vi "microFPGA_laser_mode_addr_0_ctrl.vi"(0 "VISA resource name":refnum<visa-resource-name>, 1 "laser channel":u16(ring)=3 items=["channel No 0", "channel No 1", "channel No 2", "channel No 3", "channel No 4", "channel No 5", "channel No 6", "channel No 7"], 2 "write or read":u16(ring) items=["read", "write"], 5 "Laser_mode_WRITE":u16(ring) items=["OFF", "ON", "RISING", "FALLING", "FOLLOW"], 11 "error in (no error)":errorcluster) -> (4 "VISA resource name 2":refnum<visa-resource-name>, 6 "Laser_mode_READ":u16(ring) items=["OFF", "ON", "RISING", "FALLING", "FOLLOW"], 8 "value write confirm":bool, 10 "abort_wrong_input":bool, 15 "error out":errorcluster)   [LabVIEW 2018]
panel:
  out "mode read string answer":string
  out "mode read string":string
  out "mode write string":string
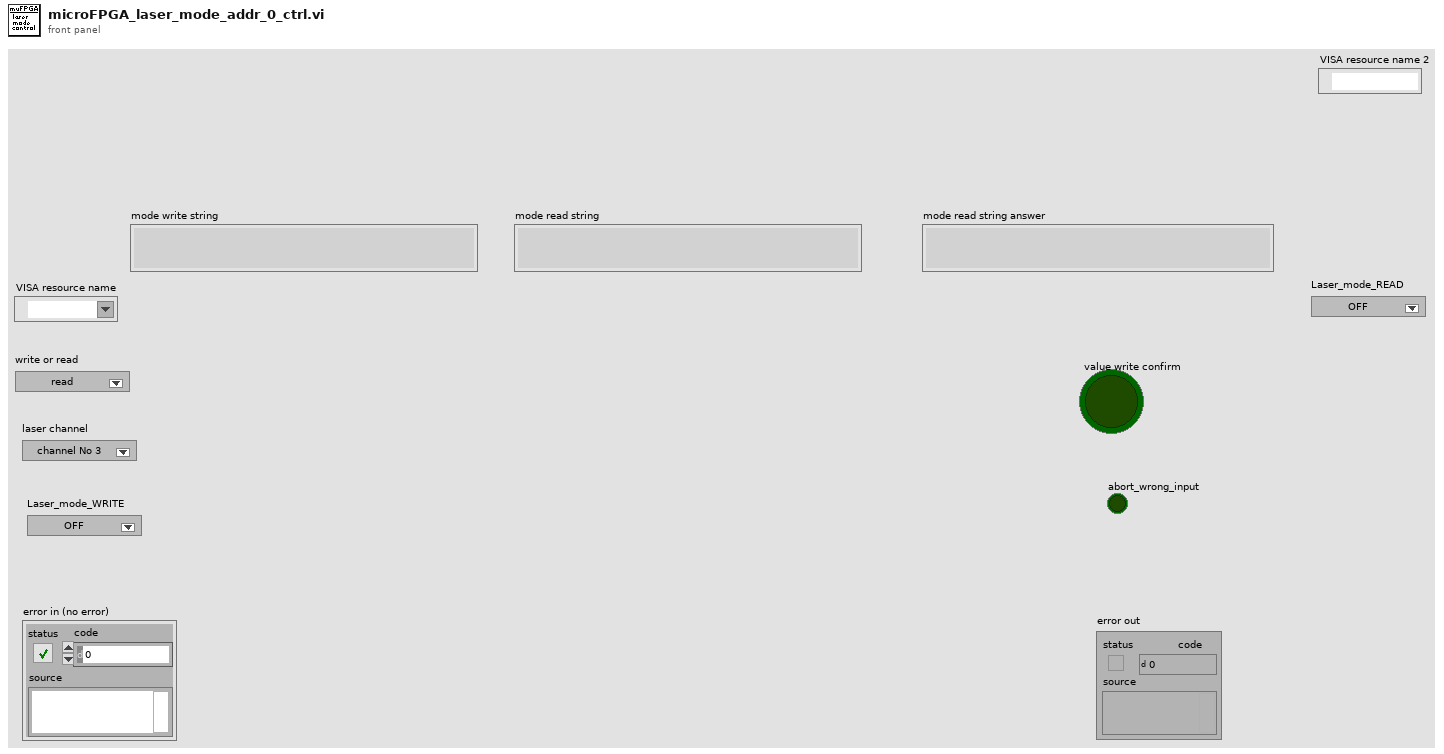
[diagram p1: front panel]
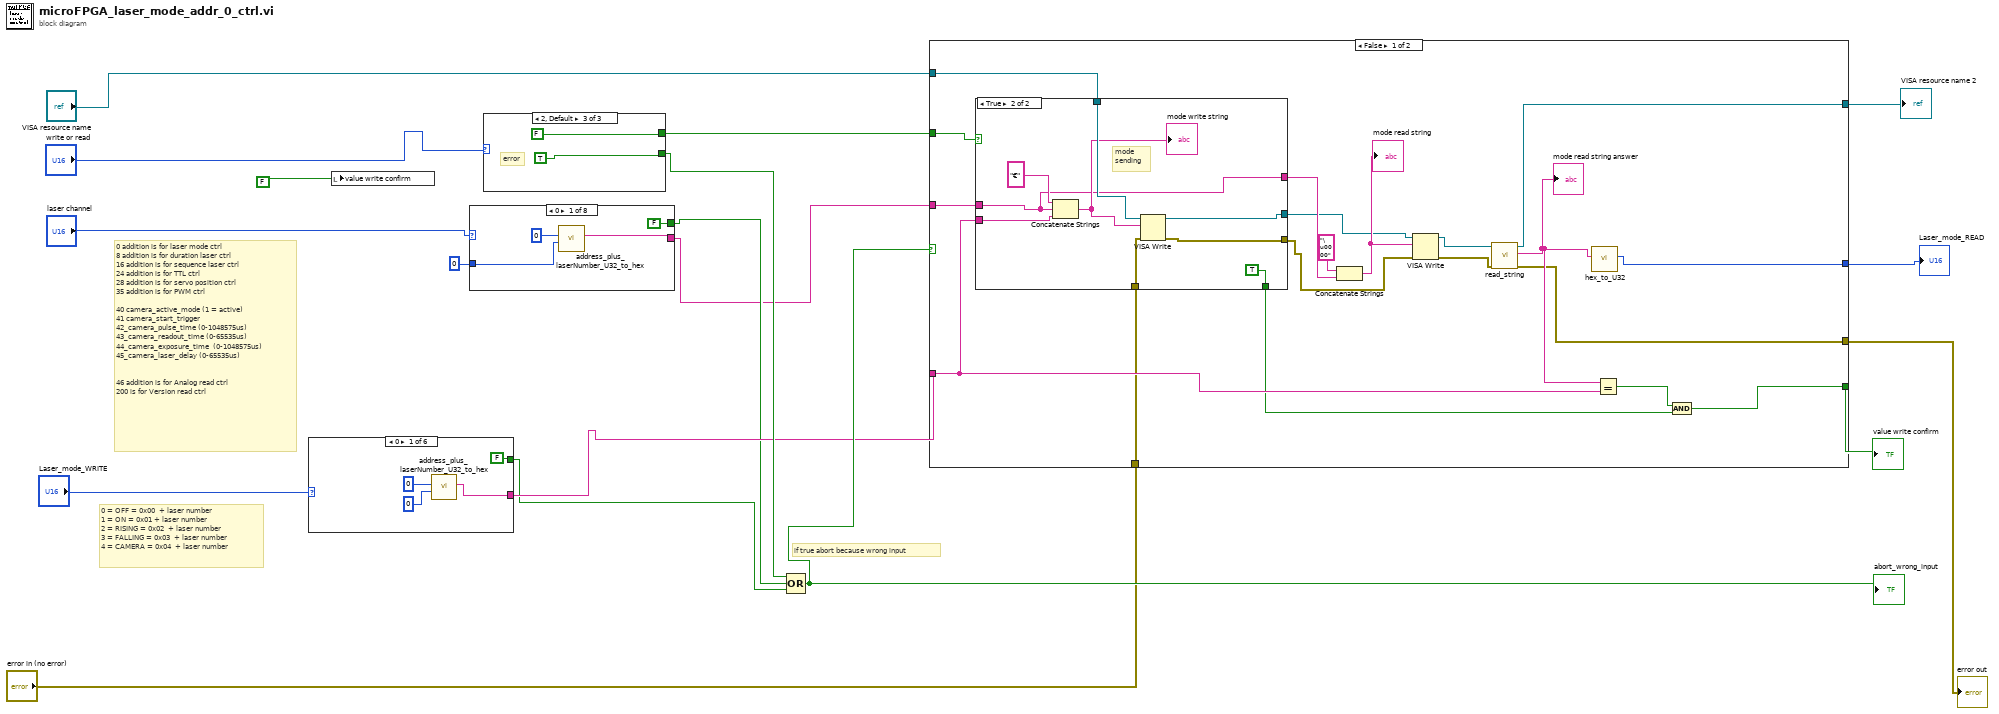
[diagram p0: block diagram]
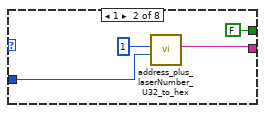
[diagram p2: hidden frame]
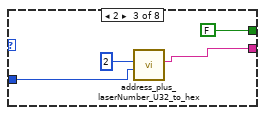
[diagram p3: hidden frame]
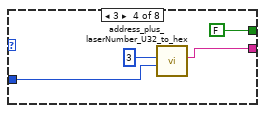
[diagram p4: hidden frame]
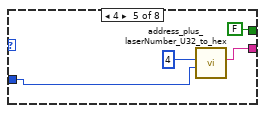
[diagram p5: hidden frame]
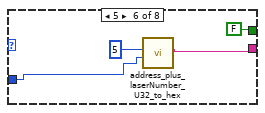
[diagram p6: hidden frame]
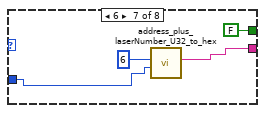
[diagram p7: hidden frame]
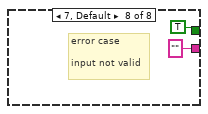
[diagram p8: hidden frame]
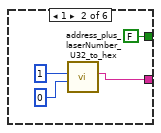
[diagram p9: hidden frame]
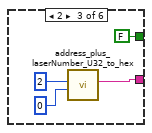
[diagram p10: hidden frame]
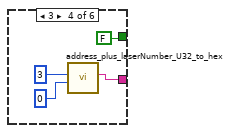
[diagram p11: hidden frame]
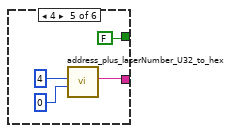
[diagram p12: hidden frame]
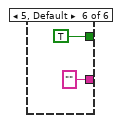
[diagram p13: hidden frame]
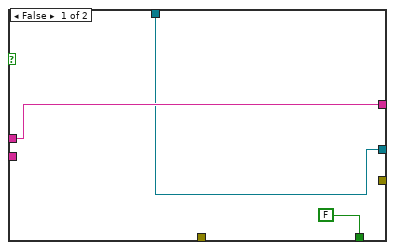
[diagram p14: hidden frame]
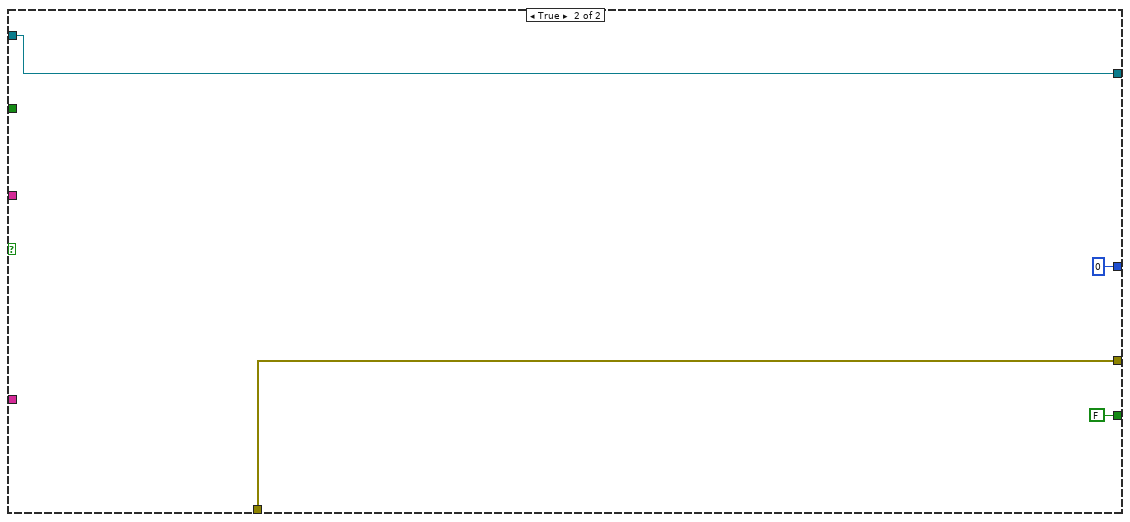
[diagram p15: hidden frame]
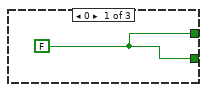
[diagram p16: hidden frame]
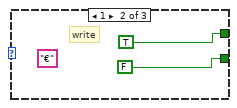
[diagram p17: hidden frame]
diagram:
  # "0 addition is for laser mode ctrl\n8 addition is for duration laser ctrl\n16 addition is for sequence laser ctrl\n24 addition is for TTL ctrl\n28 addition is for servo position ctrl\n35 addition is for PWM ctrl\n\n40 camera_active_mode (1 = active) \n41 camera_start_trigger\n42_camera_pulse_time (0-1048575us)\n43_camera_readout_time (0-65535us)\n44_camera_exposure_time  (0-1048575us)\n45_camera_laser_delay (0-65535us)\n\n\n46 addition is for Analog read ctrl\n200 is for Version read ctrl"
  # "0 = OFF = 0x00  + laser number\n1 = ON = 0x01 + laser number\n2 = RISING = 0x02  + laser number\n3 = FALLING = 0x03  + laser number\n4 = CAMERA = 0x04  + laser number"
  # "if true abort because wrong input"
  n1 = case shown="0" "Laser_mode_WRITE" {
    tunnel: [w19 w24 w28 w32 w36 "" ("string 5")] -> w7
    tunnel: [FALSE FALSE FALSE FALSE FALSE TRUE] -> w6
    frame 0 {
      n2 = call "address_plus_laserNumber_U32_to_hex.vi"("adress offset"=u32 0, "y 3"=u32 0) -> ("string 5"=w19:string)  [unwired: 8 in]
    }
    frame 1 {
      n3 = call "address_plus_laserNumber_U32_to_hex.vi"("adress offset"=u32 0, "y 3"=u32 1) -> ("string 5"=w24:string)  [unwired: 8 in]
    }
    frame 2 {
      n4 = call "address_plus_laserNumber_U32_to_hex.vi"("adress offset"=u32 0, "y 3"=u32 2) -> ("string 5"=w28:string)  [unwired: 8 in]
    }
    frame 3 {
      n5 = call "address_plus_laserNumber_U32_to_hex.vi"("adress offset"=u32 0, "y 3"=u32 3) -> ("string 5"=w32:string)  [unwired: 8 in]
    }
    frame 4 {
      n6 = call "address_plus_laserNumber_U32_to_hex.vi"("adress offset"=u32 0, "y 3"=u32 4) -> ("string 5"=w36:string)  [unwired: 8 in]
    }
    frame 5, Default {
    }
  }
  n7 = local write "value write confirm"(FALSE ("value confirm")) -> ()
  n8 = case shown="0" "laser channel" {
    tunnel: [w42 w46 w50 w54 w58 w62 w66 "" ("string 5")] -> w1
    tunnel: [FALSE FALSE FALSE FALSE FALSE FALSE FALSE TRUE] -> w2
    tunnel: u32 0 ("adress offset") -> [w41 w45 w49 w53 w57 w61 w65 _]
    frame 0 {
      n9 = call "address_plus_laserNumber_U32_to_hex.vi"("adress offset"=w41, "y 3"=u32 0) -> ("string 5"=w42:string)  [unwired: 8 in]
    }
    frame 1 {
      n10 = call "address_plus_laserNumber_U32_to_hex.vi"("adress offset"=w45, "y 3"=u32 1) -> ("string 5"=w46:string)  [unwired: 8 in]
    }
    frame 2 {
      n11 = call "address_plus_laserNumber_U32_to_hex.vi"("adress offset"=w49, "y 3"=u32 2) -> ("string 5"=w50:string)  [unwired: 8 in]
    }
    frame 3 {
      n12 = call "address_plus_laserNumber_U32_to_hex.vi"("adress offset"=w53, "y 3"=u32 3) -> ("string 5"=w54:string)  [unwired: 8 in]
    }
    frame 4 {
      n13 = call "address_plus_laserNumber_U32_to_hex.vi"("adress offset"=w57, "y 3"=u32 4) -> ("string 5"=w58:string)  [unwired: 8 in]
    }
    frame 5 {
      n14 = call "address_plus_laserNumber_U32_to_hex.vi"("adress offset"=w61, "y 3"=u32 5) -> ("string 5"=w62:string)  [unwired: 8 in]
    }
    frame 6 {
      n15 = call "address_plus_laserNumber_U32_to_hex.vi"("adress offset"=w65, "y 3"=u32 6) -> ("string 5"=w66:string)  [unwired: 8 in]
    }
    frame 7, Default {
      # "error case\n\ninput not valid"
    }
  }
  n16 = case shown="2, Default" "write or read" {
    tunnel: [w71 TRUE FALSE] -> w16
    tunnel: [w71 FALSE TRUE] -> w14
    frame 0 {
      w71 = FALSE
    }
    frame 1 {
      (unwired) "€" ("hex")
      # "write"
    }
    frame 2, Default {
      # "error"
    }
  }
  n17 = Compound Arithmetic op=OR(w14, w2, w6) -> (w12:bool)
  "abort_wrong_input" <- w12
  n18 = case shown="False" w12 {
    tunnel: "VISA resource name" -> [w94 w108]
    tunnel: w1 -> [w91 _]
    tunnel: w16 -> [w85 _]
    tunnel: w7 -> [w83 _]
    tunnel: [w82 u32 0 ("U32")] -> w5
    tunnel: [w76 FALSE] -> w13
    tunnel: [w81 w108] -> w11
    tunnel: "error in (no error)" -> [w80 w107]
    tunnel: [w79 w107] -> w9
    frame False {
      n19 = case shown="True" w85 {
        tunnel: w91 -> [w97 w103]
        tunnel: w94 -> [w96 w105]
        tunnel: [w97 w103] -> w92
        tunnel: w83 -> [_ w102]
        tunnel: [w96 w101] -> w87
        tunnel: [_ w100] -> w86
        tunnel: w80 -> [_ w99]
        tunnel: [FALSE TRUE] -> w78
        frame False {
        }
        frame True {
          # "mode \nsending"
          n20 = Concatenate Strings("€" ("string"), w103, w102) -> (w104:string)
          "mode write string" <- w104
          n21 = VISA Write(VISA resource name=w105, write buffer=w104, error in (no error)=w99) -> (VISA resource name out=w101:refnum<visa-resource-name>, error out=w100:errorcluster)  [unwired: 1 out]
        }
      }
      n22 = Concatenate Strings("\u0000" ("string"), w92) -> (w90:string)
      "mode read string" <- w90
      n23 = VISA Write(VISA resource name=w87, write buffer=w90, error in (no error)=w86) -> (VISA resource name out=w89:refnum<visa-resource-name>, error out=w88:errorcluster)  [unwired: 1 out]
      n24 = call "read_string.vi"("error in (no error)"=w88, "VISA resource name 2"=w89) -> ("error out"=w79:errorcluster, "read buffer"=w84:string, "VISA resource name"=w81:refnum<visa-resource-name>)  [unwired: 7 in]
      "mode read string answer" <- w84
      n25 = call "hex_to_U32.vi"("hex"=w84) -> ("U32"=w82:u32)  [unwired: 9 in]
      n26 = Equal?(x=w84, y=w83) -> (x = y?=w77:bool)
      n27 = And(x=w77, y=w78) -> (x .and. y?=w76:bool)
    }
    frame True {
    }
  }
  "value write confirm" <- w13
  "VISA resource name 2" <- w11
  "error out" <- w9
  "Laser_mode_READ" <- w5
